vi "trentDemo.vi"() -> ()   [LabVIEW 2011]
uses:
  <vilib>/vision/NI_Vision_Development_Module.lvlib
panel:
  out "Lines (Shape Detection 1)":T1(array[cluster]) {"End Point"."Y" format="%.2f"; "End Point"."X" format="%.2f"; "Start Point"."Y" format="%.2f"; "Start Point"."X" format="%.2f"}
  out "Image Out 2":T2(plugin-control)
  out "Luminance Plane":T2(plugin-control)
  out "Image Out":T2(plugin-control)
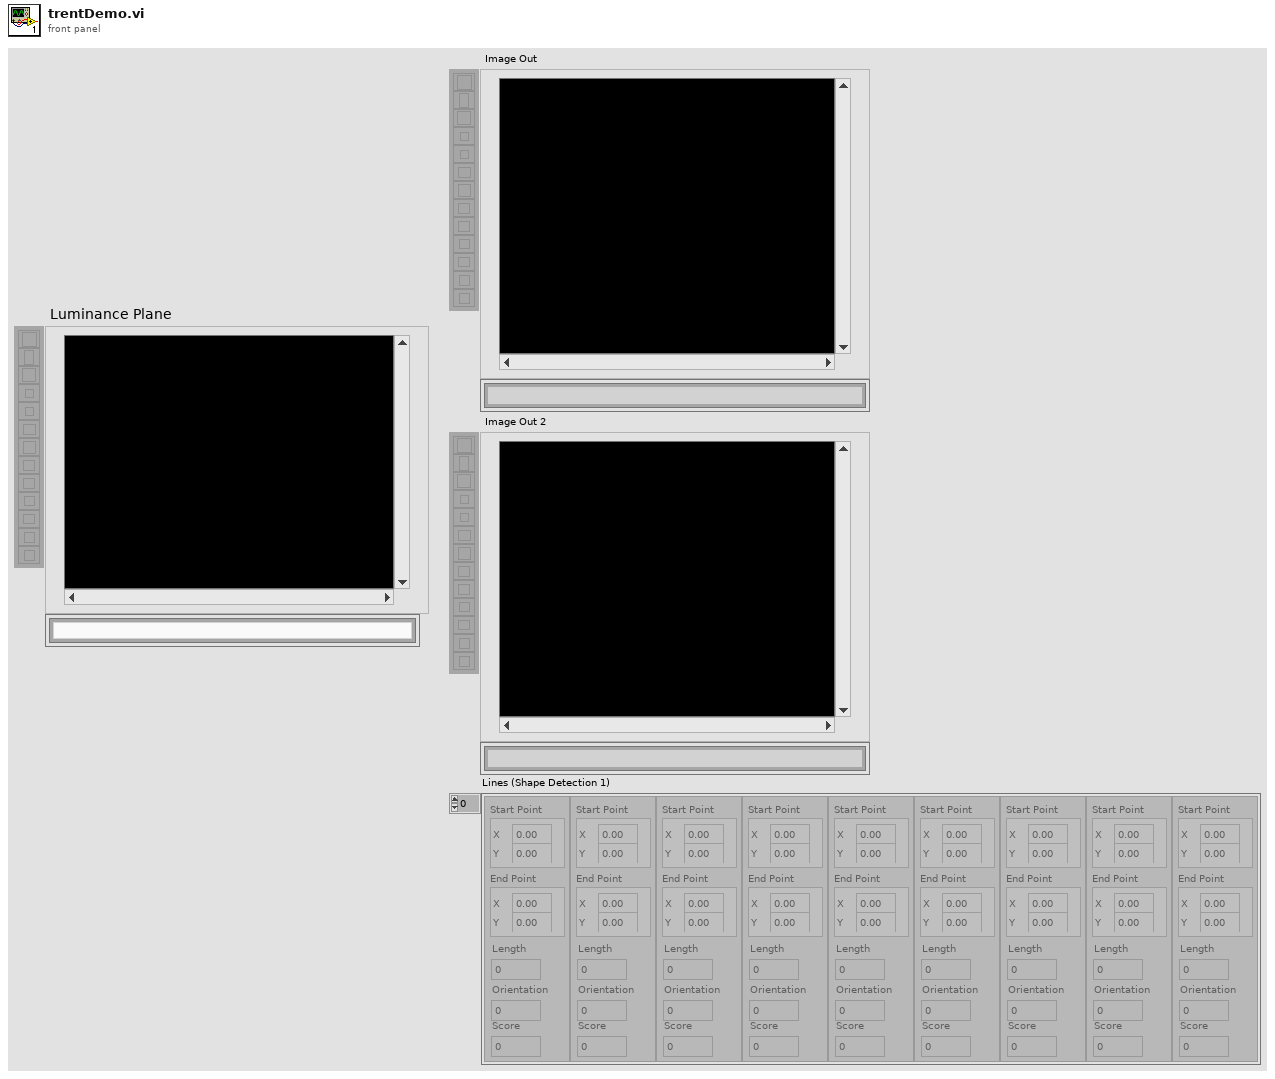
[diagram p1: front panel]
types:
  T1 = cluster{"Start Point":cluster{"X":sgl, "Y":sgl}, "End Point":cluster{"X":sgl, "Y":sgl}, "Length":dbl, "Orientation":dbl, "Score":dbl}[]
  T2 = typedef "IMAQ Image.ctl" = refnum<image>
  T3 = typedef "Image Type" = u32
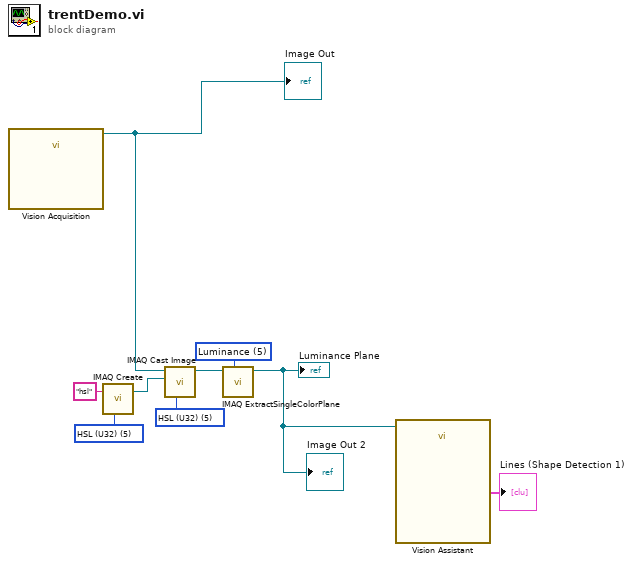
[diagram p0: block diagram]
diagram:
  w4 = 5 items=["Red", "Green", "Blue", "Hue", "Saturation", "Luminance", "Value", "Intensity"] ("Color Plane")
  w6 = T3 5 items=["Grayscale (U8)", "Grayscale (I16)", "Grayscale (SGL)", "Complex (CSG)", "RGB (U32)", "HSL (U32)", "RGB (U64)"] ("Image Type")
  w7 = T3 5 items=["Grayscale (U8)", "Grayscale (I16)", "Grayscale (SGL)", "Complex (CSG)", "RGB (U32)", "HSL (U32)", "RGB (U64)"] ("Image Type")
  n1 = call "Vision Acquisition"() -> ("Image Out"=w3:T2)  [unwired: 26 in, 1 out]
  "Image Out" <- w3
  n2 = call "IMAQ Create"("Image Name"="hsl", "Image Type"=w7) -> ("New Image"=w9:T2)  [unwired: 3 in, 1 out]
  n3 = call "IMAQ Cast Image"("Image Type"=w6, "Image Dst"=w9, "Image Src"=w3) -> ("Image Dst Out"=w5:T2)  [unwired: 7 in, 1 out]
  n4 = call "IMAQ ExtractSingleColorPlane"("Color Plane"=w4, "Image Src"=w5) -> ("Image Dst Out"=w2:T2)  [unwired: 8 in, 1 out]
  "Luminance Plane" <- w2
  "Image Out 2" <- w2
  n5 = call "Vision Assistant"("Image In"=w2) -> ("Lines (Shape Detection 1)"=→"Lines (Shape Detection 1)":T1)  [unwired: 22 in, 4 out]
